vi "Register gRPC Messages.vi"(8 "error in (no error)":errorcluster, 11 "gRPC ID":T1) -> (0 "error out":errorcluster, 3 "gRPC ID Out":T1)   [LabVIEW 2020, in "FlexLogger_client.lvlib"]
uses:
  FlexLogger_client.lvlib
  <vilib>/gRPC/LabVIEW gRPC Library/Shared/grpcId.ctl
  <vilib>/gRPC/LabVIEW gRPC Library/Server API/typeDefs/Message Metadata.ctl
  <vilib>/gRPC/LabVIEW gRPC Library/Server API/typeDefs/Message Element Metadata.ctl
  <vilib>/gRPC/LabVIEW gRPC Library/Server API/typeDefs/Message Element Type.ctl
  <vilib>/gRPC/LabVIEW gRPC Library/grpc-lvsupport-release.lvlib
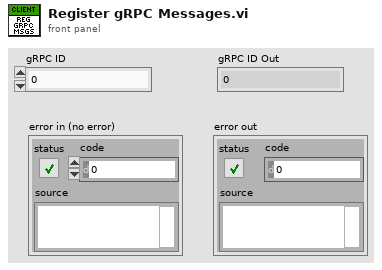
[diagram p1: front panel]
types:
  T1 = typedef "grpc-lvsupport-release.lvlib/grpcId.ctl" = u64
  T2 = typedef "grpc-lvsupport-release.lvlib/Message Metadata.ctl" = cluster{"Version":i32, "Name":string, "Type Url":string, "Elements":T3[]}
  T3 = typedef "grpc-lvsupport-release.lvlib/Message Element Metadata.ctl" = cluster{"Embedded Message Name":string, "Protobuf Index":i32, "MessageElementType":T4, "Repeated":bool}
  T4 = typedef "grpc-lvsupport-release.lvlib/Message Element Type.ctl" = enum32{"Int32Value", "FloatValue", "DoubleValue", "BoolValue", "StringValue", "MessageValue", "Int64Value", "UInt32Value", "UInt64Value", "EnumValue", "Bytes", "Fixed64", "Fixed32", "SFixed64", "SFixed32", "SInt64", "SInt32"}
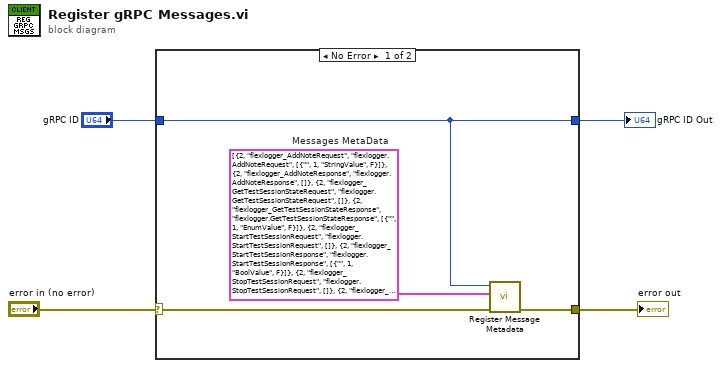
[diagram p0: block diagram]
diagram:
  n1 = case shown="No Error" "error in (no error)" {
    selector: "error in (no error)" -> [w6 w10]
    tunnel: [w5 w9] -> w1
    tunnel: [w8 w10] -> w4
    tunnel: "gRPC ID" -> [w5 w9]
    frame No Error {
      w7 = T2[] [{"Version"=2, "Name"="flexlogger_AddNoteRequest", "Type Url"="flexlogger.AddNoteRequest", "Elements"=[{"Embedded Message Name"="", "Protobuf Index"=1, "MessageElementType"=enum."StringValue", "Repeated"=FALSE}]}, {"Version"=2, "Name"="flexlogger_AddNoteResponse", "Type Url"="flexlogger.AddNoteResponse", "Elements"=[]}, {"Version"=2, "Name"="flexlogger_GetTestSessionStateRequest", "Type Url"="flexlogger.GetTestSessionStateRequest", "Elements"=[]}, {"Version"=2, "Name"="flexlogger_GetTestSessionStateResponse", "Type Url"="flexlogger.GetTestSessionStateResponse", "Elements"=[{"Embedded Message Name"="", "Protobuf Index"=1, "MessageElementType"=enum."EnumValue", "Repeated"=FALSE}]}, {"Version"=2, "Name"="flexlogger_StartTestSessionRequest", "Type Url"="flexlogger.StartTestSessionRequest", "Elements"=[]}, {"Version"=2, "Name"="flexlogger_StartTestSessionResponse", "Type Url"="flexlogger.StartTestSessionResponse", "Elements"=[{"Embedded Message Name"="", "Protobuf Index"=1, "MessageElementType"=enum."BoolValue", "Repeated"=FALSE}]}, {"Version"=2, "Name"="flexlogger_StopTestSessionRequest", "Type Url"="flexlogger.StopTestSessionRequest", "Elements"=[]}, {"Version"=2, "Name"="flexlogger_StopTestSessionResponse", "Type Url"="flexlogger.StopTestSessionResponse", "Elements"=[{"Embedded Message Name"="", "Protobuf Index"=1, "MessageElementType"=enum."BoolValue", "Repeated"=FALSE}]}, {"Version"=2, "Name"="flexlogger_PauseTestSessionRequest", "Type Url"="flexlogger.PauseTestSessionRequest", "Elements"=[]}, {"Version"=2, "Name"="flexlogger_PauseTestSessionResponse", "Type Url"="flexlogger.PauseTestSessionResponse", "Elements"=[{"Embedded Message Name"="", "Protobuf Index"=1, "MessageElementType"=enum."BoolValue", "Repeated"=FALSE}]}, {"Version"=2, "Name"="flexlogger_ResumeTestSessionRequest", "Type Url"="flexlogger.ResumeTestSessionRequest", "Elements"=[]}, {"Version"=2, "Name"="flexlogger_ResumeTestSessionResponse", "Type Url"="flexlogger.ResumeTestSessionResponse", "Elements"=[{"Embedded Message Name"="", "Protobuf Index"=1, "MessageElementType"=enum."BoolValue", "Repeated"=FALSE}]}, {"Version"=2, "Name"="flexlogger_GetElapsedTestTimeRequest", "Type Url"="flexlogger.GetElapsedTestTimeRequest", "Elements"=[]}, {"Version"=2, "Name"="flexlogger_GetElapsedTestTimeResponse", "Type Url"="flexlogger.GetElapsedTestTimeResponse", "Elements"=[{"Embedded Message Name"="", "Protobuf Index"=1, "MessageElementType"=enum."DoubleValue", "Repeated"=FALSE}]}, {"Version"=2, "Name"="flexlogger_GetLogFileDescriptionRequest", "Type Url"="flexlogger.GetLogFileDescriptionRequest", "Elements"=[{"Embedded Message Name"="flexlogger_ElementIdentifier", "Protobuf Index"=1, "MessageElementType"=enum."MessageValue", "Repeated"=FALSE}]}, {"Version"=2, "Name"="flexlogger_GetLogFileDescriptionResponse", "Type Url"="flexlogger.GetLogFileDescriptionResponse", "Elements"=[{"Embedded Message Name"="", "Protobuf Index"=1, "MessageElementType"=enum."StringValue", "Repeated"=FALSE}]}, {"Version"=2, "Name"="flexlogger_SetLogFileDescriptionRequest", "Type Url"="flexlogger.SetLogFileDescriptionRequest", "Elements"=[{"Embedded Message Name"="flexlogger_ElementIdentifier", "Protobuf Index"=1, "MessageElementType"=enum."MessageValue", "Repeated"=FALSE}, {"Embedded Message Name"="", "Protobuf Index"=2, "MessageElementType"=enum."StringValue", "Repeated"=FALSE}]}, {"Version"=2, "Name"="flexlogger_SetTestPropertiesRequest", "Type Url"="flexlogger.SetTestPropertiesRequest", "Elements"=[{"Embedded Message Name"="flexlogger_ElementIdentifier", "Protobuf Index"=1, "MessageElementType"=enum."MessageValue", "Repeated"=FALSE}, {"Embedded Message Name"="flexlogger_TestProperty", "Protobuf Index"=2, "MessageElementType"=enum."MessageValue", "Repeated"=TRUE}]}, {"Version"=2, "Name"="flexlogger_GetLogFileBasePathRequest", "Type Url"="flexlogger.GetLogFileBasePathRequest", "Elements"=[{"Embedded Message Name"="flexlogger_ElementIdentifier", "Protobuf Index"=1, "MessageElementType"=enum."MessageValue", "Repeated"=FALSE}]}, {"Version"=2, "Name"="flexlogger_GetLogFileBasePathResponse", "Type Url"="flexlogger.GetLogFileBasePathResponse", "Elements"=[{"Embedded Message Name"="", "Protobuf Index"=1, "MessageElementType"=enum."StringValue", "Repeated"=FALSE}]}, {"Version"=2, "Name"="flexlogger_SetLogFileBasePathRequest", "Type Url"="flexlogger.SetLogFileBasePathRequest", "Elements"=[{"Embedded Message Name"="flexlogger_ElementIdentifier", "Protobuf Index"=1, "MessageElementType"=enum."MessageValue", "Repeated"=FALSE}, {"Embedded Message Name"="", "Protobuf Index"=2, "MessageElementType"=enum."StringValue", "Repeated"=FALSE}]}, {"Version"=2, "Name"="flexlogger_SetLogFileBasePathResponse", "Type Url"="flexlogger.SetLogFileBasePathResponse", "Elements"=[]}, {"Version"=2, "Name"="flexlogger_GetLogFileNameRequest", "Type Url"="flexlogger.GetLogFileNameRequest", "Elements"=[{"Embedded Message Name"="flexlogger_ElementIdentifier", "Protobuf Index"=1, "MessageElementType"=enum."MessageValue", "Repeated"=FALSE}]}, {"Version"=2, "Name"="flexlogger_GetLogFileNameResponse", "Type Url"="flexlogger.GetLogFileNameResponse", "Elements"=[{"Embedded Message Name"="", "Protobuf Index"=1, "MessageElementType"=enum."StringValue", "Repeated"=FALSE}]}, {"Version"=2, "Name"="flexlogger_SetLogFileNameRequest", "Type Url"="flexlogger.SetLogFileNameRequest", "Elements"=[{"Embedded Message Name"="flexlogger_ElementIdentifier", "Protobuf Index"=1, "MessageElementType"=enum."MessageValue", "Repeated"=FALSE}, {"Embedded Message Name"="", "Protobuf Index"=2, "MessageElementType"=enum."StringValue", "Repeated"=FALSE}]}, {"Version"=2, "Name"="flexlogger_SetLogFileNameResponse", "Type Url"="flexlogger.SetLogFileNameResponse", "Elements"=[]}, {"Version"=2, "Name"="flexlogger_TestProperty", "Type Url"="flexlogger.TestProperty", "Elements"=[{"Embedded Message Name"="", "Protobuf Index"=1, "MessageElementType"=enum."StringValue", "Repeated"=FALSE}, {"Embedded Message Name"="", "Protobuf Index"=2, "MessageElementType"=enum."StringValue", "Repeated"=FALSE}, {"Embedded Message Name"="", "Protobuf Index"=3, "MessageElementType"=enum."BoolValue", "Repeated"=FALSE}]}, {"Version"=2, "Name"="flexlogger_GetTestPropertiesRequest", "Type Url"="flexlogger.GetTestPropertiesRequest", "Elements"=[{"Embedded Message Name"="flexlogger_ElementIdentifier", "Protobuf Index"=1, "MessageElementType"=enum."MessageValue", "Repeated"=FALSE}]}, {"Version"=2, "Name"="flexlogger_GetTestPropertiesResponse", "Type Url"="flexlogger.GetTestPropertiesResponse", "Elements"=[{"Embedded Message Name"="flexlogger_TestProperty", "Protobuf Index"=1, "MessageElementType"=enum."MessageValue", "Repeated"=TRUE}]}, {"Version"=2, "Name"="flexlogger_GetTestPropertyRequest", "Type Url"="flexlogger.GetTestPropertyRequest", "Elements"=[{"Embedded Message Name"="flexlogger_ElementIdentifier", "Protobuf Index"=1, "MessageElementType"=enum."MessageValue", "Repeated"=FALSE}, {"Embedded Message Name"="", "Protobuf Index"=2, "MessageElementType"=enum."StringValue", "Repeated"=FALSE}]}, {"Version"=2, "Name"="flexlogger_GetTestPropertyResponse", "Type Url"="flexlogger.GetTestPropertyResponse", "Elements"=[{"Embedded Message Name"="flexlogger_TestProperty", "Protobuf Index"=1, "MessageElementType"=enum."MessageValue", "Repeated"=FALSE}]}, {"Version"=2, "Name"="flexlogger_SetTestPropertyRequest", "Type Url"="flexlogger.SetTestPropertyRequest", "Elements"=[{"Embedded Message Name"="flexlogger_ElementIdentifier", "Protobuf Index"=1, "MessageElementType"=enum."MessageValue", "Repeated"=FALSE}, {"Embedded Message Name"="flexlogger_TestProperty", "Protobuf Index"=2, "MessageElementType"=enum."MessageValue", "Repeated"=FALSE}]}, {"Version"=2, "Name"="flexlogger_SetTestPropertyResponse", "Type Url"="flexlogger.SetTestPropertyResponse", "Elements"=[]}, {"Version"=2, "Name"="flexlogger_RemoveTestPropertyRequest", "Type Url"="flexlogger.RemoveTestPropertyRequest", "Elements"=[{"Embedded Message Name"="flexlogger_ElementIdentifier", "Protobuf Index"=1, "MessageElementType"=enum."MessageValue", "Repeated"=FALSE}, {"Embedded Message Name"="", "Protobuf Index"=2, "MessageElementType"=enum."StringValue", "Repeated"=FALSE}]}, {"Version"=2, "Name"="flexlogger_RemoveTestPropertyResponse", "Type Url"="flexlogger.RemoveTestPropertyResponse", "Elements"=[]}, {"Version"=2, "Name"="flexlogger_GetResolvedLogFileBasePathRequest", "Type Url"="flexlogger.GetResolvedLogFileBasePathRequest", "Elements"=[{"Embedded Message Name"="flexlogger_ElementIdentifier", "Protobuf Index"=1, "MessageElementType"=enum."MessageValue", "Repeated"=FALSE}]}, {"Version"=2, "Name"="flexlogger_GetResolvedLogFileBasePathResponse", "Type Url"="flexlogger.GetResolvedLogFileBasePathResponse", "Elements"=[{"Embedded Message Name"="", "Protobuf Index"=1, "MessageElementType"=enum."StringValue", "Repeated"=FALSE}]}, {"Version"=2, "Name"="flexlogger_GetResolvedLogFileNameRequest", "Type Url"="flexlogger.GetResolvedLogFileNameRequest", "Elements"=[{"Embedded Message Name"="flexlogger_ElementIdentifier", "Protobuf Index"=1, "MessageElementType"=enum."MessageValue", "Repeated"=FALSE}]}, {"Version"=2, "Name"="flexlogger_GetResolvedLogFileNameResponse", "Type Url"="flexlogger.GetResolvedLogFileNameResponse", "Elements"=[{"Embedded Message Name"="", "Protobuf Index"=1, "MessageElementType"=enum."StringValue", "Repeated"=FALSE}]}, {"Version"=2, "Name"="flexlogger_ProjectIdentifier", "Type Url"="flexlogger.ProjectIdentifier", "Elements"=[{"Embedded Message Name"="", "Protobuf Index"=1, "MessageElementType"=enum."StringValue", "Repeated"=FALSE}]}, {"Version"=2, "Name"="flexlogger_ElementIdentifier", "Type Url"="flexlogger.ElementIdentifier", "Elements"=[{"Embedded Message Name"="", "Protobuf Index"=1, "MessageElementType"=enum."StringValue", "Repeated"=FALSE}, {"Embedded Message Name"="", "Protobuf Index"=2, "MessageElementType"=enum."StringValue", "Repeated"=FALSE}, {"Embedded Message Name"="", "Protobuf Index"=3, "MessageElementType"=enum."StringValue", "Repeated"=FALSE}, {"Embedded Message Name"="", "Protobuf Index"=4, "MessageElementType"=enum."StringValue", "Repeated"=FALSE}]}, {"Version"=2, "Name"="flexlogger_ConnectRequest", "Type Url"="flexlogger.ConnectRequest", "Elements"=[]}, {"Version"=2, "Name"="flexlogger_ConnectResponse", "Type Url"="flexlogger.ConnectResponse", "Elements"=[]}, {"Version"=2, "Name"="flexlogger_DisconnectRequest", "Type Url"="flexlogger.DisconnectRequest", "Elements"=[{"Embedded Message Name"="", "Protobuf Index"=1, "MessageElementType"=enum."BoolValue", "Repeated"=FALSE}]}, {"Version"=2, "Name"="flexlogger_DisconnectResponse", "Type Url"="flexlogger.DisconnectResponse", "Elements"=[]}, {"Version"=2, "Name"="flexlogger_GetPreferencesDirectoryRequest", "Type Url"="flexlogger.GetPreferencesDirectoryRequest", "Elements"=[]}, {"Version"=2, "Name"="flexlogger_GetPreferencesDirectoryResponse", "Type Url"="flexlogger.GetPreferencesDirectoryResponse", "Elements"=[{"Embedded Message Name"="", "Protobuf Index"=1, "MessageElementType"=enum."StringValue", "Repeated"=FALSE}]}, {"Version"=2, "Name"="flexlogger_OpenProjectRequest", "Type Url"="flexlogger.OpenProjectRequest", "Elements"=[{"Embedded Message Name"="", "Protobuf Index"=1, "MessageElementType"=enum."StringValue", "Repeated"=FALSE}]}, {"Version"=2, "Name"="flexlogger_OpenProjectResponse", "Type Url"="flexlogger.OpenProjectResponse", "Elements"=[{"Embedded Message Name"="flexlogger_ProjectIdentifier", "Protobuf Index"=1, "MessageElementType"=enum."MessageValue", "Repeated"=FALSE}]}, {"Version"=2, "Name"="flexlogger_GetActiveProjectRequest", "Type Url"="flexlogger.GetActiveProjectRequest", "Elements"=[]}, {"Version"=2, "Name"="flexlogger_GetActiveProjectResponse", "Type Url"="flexlogger.GetActiveProjectResponse", "Elements"=[{"Embedded Message Name"="", "Protobuf Index"=1, "MessageElementType"=enum."BoolValue", "Repeated"=FALSE}, {"Embedded Message Name"="flexlogger_ProjectIdentifier", "Protobuf Index"=2, "MessageElementType"=enum."MessageValue", "Repeated"=FALSE}]}, {"Version"=2, "Name"="flexlogger_Empty", "Type Url"="flexlogger.Empty", "Elements"=[]}, {"Version"=2, "Name"="flexlogger_OpenChannelSpecificationDocumentRequest", "Type Url"="flexlogger.OpenChannelSpecificationDocumentRequest", "Elements"=[{"Embedded Message Name"="flexlogger_ProjectIdentifier", "Protobuf Index"=1, "MessageElementType"=enum."MessageValue", "Repeated"=FALSE}]}, {"Version"=2, "Name"="flexlogger_OpenChannelSpecificationDocumentResponse", "Type Url"="flexlogger.OpenChannelSpecificationDocumentResponse", "Elements"=[{"Embedded Message Name"="flexlogger_ElementIdentifier", "Protobuf Index"=1, "MessageElementType"=enum."MessageValue", "Repeated"=FALSE}]}, {"Version"=2, "Name"="flexlogger_OpenLoggingSpecificationDocumentRequest", "Type Url"="flexlogger.OpenLoggingSpecificationDocumentRequest", "Elements"=[{"Embedded Message Name"="flexlogger_ProjectIdentifier", "Protobuf Index"=1, "MessageElementType"=enum."MessageValue", "Repeated"=FALSE}]}, {"Version"=2, "Name"="flexlogger_OpenLoggingSpecificationDocumentResponse", "Type Url"="flexlogger.OpenLoggingSpecificationDocumentResponse", "Elements"=[{"Embedded Message Name"="flexlogger_ElementIdentifier", "Protobuf Index"=1, "MessageElementType"=enum."MessageValue", "Repeated"=FALSE}]}, {"Version"=2, "Name"="flexlogger_OpenScreenDocumentRequest", "Type Url"="flexlogger.OpenScreenDocumentRequest", "Elements"=[{"Embedded Message Name"="flexlogger_ProjectIdentifier", "Protobuf Index"=1, "MessageElementType"=enum."MessageValue", "Repeated"=FALSE}, {"Embedded Message Name"="", "Protobuf Index"=2, "MessageElementType"=enum."StringValue", "Repeated"=FALSE}]}, {"Version"=2, "Name"="flexlogger_OpenScreenDocumentResponse", "Type Url"="flexlogger.OpenScreenDocumentResponse", "Elements"=[{"Embedded Message Name"="flexlogger_ElementIdentifier", "Protobuf Index"=1, "MessageElementType"=enum."MessageValue", "Repeated"=FALSE}]}, {"Version"=2, "Name"="flexlogger_OpenTestSpecificationDocumentRequest", "Type Url"="flexlogger.OpenTestSpecificationDocumentRequest", "Elements"=[{"Embedded Message Name"="flexlogger_ProjectIdentifier", "Protobuf Index"=1, "MessageElementType"=enum."MessageValue", "Repeated"=FALSE}]}, {"Version"=2, "Name"="flexlogger_OpenTestSpecificationDocumentResponse", "Type Url"="flexlogger.OpenTestSpecificationDocumentResponse", "Elements"=[{"Embedded Message Name"="flexlogger_ElementIdentifier", "Protobuf Index"=1, "MessageElementType"=enum."MessageValue", "Repeated"=FALSE}]}, {"Version"=2, "Name"="flexlogger_CloseProjectRequest", "Type Url"="flexlogger.CloseProjectRequest", "Elements"=[{"Embedded Message Name"="", "Protobuf Index"=1, "MessageElementType"=enum."BoolValue", "Repeated"=FALSE}]}, {"Version"=2, "Name"="flexlogger_CloseProjectResponse", "Type Url"="flexlogger.CloseProjectResponse", "Elements"=[]}, {"Version"=2, "Name"="flexlogger_GetProjectFilePathRequest", "Type Url"="flexlogger.GetProjectFilePathRequest", "Elements"=[{"Embedded Message Name"="flexlogger_ProjectIdentifier", "Protobuf Index"=1, "MessageElementType"=enum."MessageValue", "Repeated"=FALSE}]}, {"Version"=2, "Name"="flexlogger_GetProjectFilePathResponse", "Type Url"="flexlogger.GetProjectFilePathResponse", "Elements"=[{"Embedded Message Name"="", "Protobuf Index"=1, "MessageElementType"=enum."StringValue", "Repeated"=FALSE}]}, {"Version"=2, "Name"="flexlogger_GetChannelNamesRequest", "Type Url"="flexlogger.GetChannelNamesRequest", "Elements"=[{"Embedded Message Name"="flexlogger_ElementIdentifier", "Protobuf Index"=1, "MessageElementType"=enum."MessageValue", "Repeated"=FALSE}]}, {"Version"=2, "Name"="flexlogger_GetChannelNamesResponse", "Type Url"="flexlogger.GetChannelNamesResponse", "Elements"=[{"Embedded Message Name"="", "Protobuf Index"=1, "MessageElementType"=enum."StringValue", "Repeated"=TRUE}]}, {"Version"=2, "Name"="flexlogger_GetDoubleChannelValueRequest", "Type Url"="flexlogger.GetDoubleChannelValueRequest", "Elements"=[{"Embedded Message Name"="flexlogger_ElementIdentifier", "Protobuf Index"=1, "MessageElementType"=enum."MessageValue", "Repeated"=FALSE}, {"Embedded Message Name"="", "Protobuf Index"=2, "MessageElementType"=enum."StringValue", "Repeated"=FALSE}]}, {"Version"=2, "Name"="flexlogger_GetDoubleChannelValueResponse", "Type Url"="flexlogger.GetDoubleChannelValueResponse", "Elements"=[{"Embedded Message Name"="flexlogger_Timestamp", "Protobuf Index"=1, "MessageElementType"=enum."MessageValue", "Repeated"=FALSE}, {"Embedded Message Name"="", "Protobuf Index"=2, "MessageElementType"=enum."DoubleValue", "Repeated"=FALSE}]}, {"Version"=2, "Name"="flexlogger_SetDoubleChannelValueRequest", "Type Url"="flexlogger.SetDoubleChannelValueRequest", "Elements"=[{"Embedded Message Name"="flexlogger_ElementIdentifier", "Protobuf Index"=1, "MessageElementType"=enum."MessageValue", "Repeated"=FALSE}, {"Embedded Message Name"="", "Protobuf Index"=2, "MessageElementType"=enum."StringValue", "Repeated"=FALSE}, {"Embedded Message Name"="", "Protobuf Index"=3, "MessageElementType"=enum."DoubleValue", "Repeated"=FALSE}]}, {"Version"=2, "Name"="flexlogger_SetDoubleChannelValueResponse", "Type Url"="flexlogger.SetDoubleChannelValueResponse", "Elements"=[]}, {"Version"=2, "Name"="flexlogger_IsChannelEnabledRequest", "Type Url"="flexlogger.IsChannelEnabledRequest", "Elements"=[{"Embedded Message Name"="flexlogger_ElementIdentifier", "Protobuf Index"=1, "MessageElementType"=enum."MessageValue", "Repeated"=FALSE}, {"Embedded Message Name"="", "Protobuf Index"=2, "MessageElementType"=enum."StringValue", "Repeated"=FALSE}]}, {"Version"=2, "Name"="flexlogger_IsChannelEnabledResponse", "Type Url"="flexlogger.IsChannelEnabledResponse", "Elements"=[{"Embedded Message Name"="", "Protobuf Index"=1, "MessageElementType"=enum."BoolValue", "Repeated"=FALSE}]}, {"Version"=2, "Name"="flexlogger_SetChannelEnabledRequest", "Type Url"="flexlogger.SetChannelEnabledRequest", "Elements"=[{"Embedded Message Name"="flexlogger_ElementIdentifier", "Protobuf Index"=1, "MessageElementType"=enum."MessageValue", "Repeated"=FALSE}, {"Embedded Message Name"="", "Protobuf Index"=2, "MessageElementType"=enum."StringValue", "Repeated"=FALSE}, {"Embedded Message Name"="", "Protobuf Index"=3, "MessageElementType"=enum."BoolValue", "Repeated"=FALSE}]}, {"Version"=2, "Name"="flexlogger_SetChannelEnabledResponse", "Type Url"="flexlogger.SetChannelEnabledResponse", "Elements"=[]}, {"Version"=2, "Name"="flexlogger_GetDataRateRequest", "Type Url"="flexlogger.GetDataRateRequest", "Elements"=[{"Embedded Message Name"="flexlogger_ElementIdentifier", "Protobuf Index"=1, "MessageElementType"=enum."MessageValue", "Repeated"=FALSE}, {"Embedded Message Name"="", "Protobuf Index"=2, "MessageElementType"=enum."EnumValue", "Repeated"=FALSE}]}, {"Version"=2, "Name"="flexlogger_GetDataRateResponse", "Type Url"="flexlogger.GetDataRateResponse", "Elements"=[{"Embedded Message Name"="", "Protobuf Index"=1, "MessageElementType"=enum."DoubleValue", "Repeated"=FALSE}]}, {"Version"=2, "Name"="flexlogger_SetDataRateRequest", "Type Url"="flexlogger.SetDataRateRequest", "Elements"=[{"Embedded Message Name"="flexlogger_ElementIdentifier", "Protobuf Index"=1, "MessageElementType"=enum."MessageValue", "Repeated"=FALSE}, {"Embedded Message Name"="", "Protobuf Index"=2, "MessageElementType"=enum."EnumValue", "Repeated"=FALSE}, {"Embedded Message Name"="", "Protobuf Index"=3, "MessageElementType"=enum."DoubleValue", "Repeated"=FALSE}]}, {"Version"=2, "Name"="flexlogger_GetDataRateLevelRequest", "Type Url"="flexlogger.GetDataRateLevelRequest", "Elements"=[{"Embedded Message Name"="flexlogger_ElementIdentifier", "Protobuf Index"=1, "MessageElementType"=enum."MessageValue", "Repeated"=FALSE}, {"Embedded Message Name"="", "Protobuf Index"=2, "MessageElementType"=enum."StringValue", "Repeated"=FALSE}]}, {"Version"=2, "Name"="flexlogger_GetDataRateLevelResponse", "Type Url"="flexlogger.GetDataRateLevelResponse", "Elements"=[{"Embedded Message Name"="", "Protobuf Index"=1, "MessageElementType"=enum."EnumValue", "Repeated"=FALSE}]}, {"Version"=2, "Name"="flexlogger_SetDataRateLevelRequest", "Type Url"="flexlogger.SetDataRateLevelRequest", "Elements"=[{"Embedded Message Name"="flexlogger_ElementIdentifier", "Protobuf Index"=1, "MessageElementType"=enum."MessageValue", "Repeated"=FALSE}, {"Embedded Message Name"="", "Protobuf Index"=2, "MessageElementType"=enum."StringValue", "Repeated"=FALSE}, {"Embedded Message Name"="", "Protobuf Index"=3, "MessageElementType"=enum."EnumValue", "Repeated"=FALSE}]}, {"Version"=2, "Name"="flexlogger_GetActualDataRateRequest", "Type Url"="flexlogger.GetActualDataRateRequest", "Elements"=[{"Embedded Message Name"="flexlogger_ElementIdentifier", "Protobuf Index"=1, "MessageElementType"=enum."MessageValue", "Repeated"=FALSE}, {"Embedded Message Name"="", "Protobuf Index"=2, "MessageElementType"=enum."StringValue", "Repeated"=FALSE}]}, {"Version"=2, "Name"="flexlogger_GetActualDataRateResponse", "Type Url"="flexlogger.GetActualDataRateResponse", "Elements"=[{"Embedded Message Name"="", "Protobuf Index"=1, "MessageElementType"=enum."DoubleValue", "Repeated"=FALSE}]}, {"Version"=2, "Name"="flexlogger_Timestamp", "Type Url"="flexlogger.Timestamp", "Elements"=[{"Embedded Message Name"="", "Protobuf Index"=1, "MessageElementType"=enum."Int64Value", "Repeated"=FALSE}, {"Embedded Message Name"="", "Protobuf Index"=2, "MessageElementType"=enum."Int32Value", "Repeated"=FALSE}]}]  # Messages MetaData
      n2 = call <vilib>:"Register Message Metadata.vi"("error in"=w6, "Messages"=w7, "gRPCid in"=w5) -> ("error out"=w8:errorcluster)  [unwired: 7 in, 1 out]
    }
    frame Error {
    }
  }
  "error out" <- w4
  "gRPC ID Out" <- w1
